vi "Read Lockinsens.vi"(1 "VISA resource name":refnum<visa-resource-name>="COM12", 2 "Voltage(T) Current(F)":bool=TRUE) -> (0 "Sensitivity":dbl=1e-08)   [LabVIEW 2013]
uses:
  <vilib>/Instr/_visa.llb/VISA Configure Serial Port (Instr).vi
panel:
  in  "milliseconds to wait":u32=50
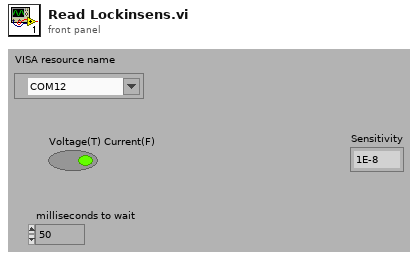
[diagram p1: front panel]
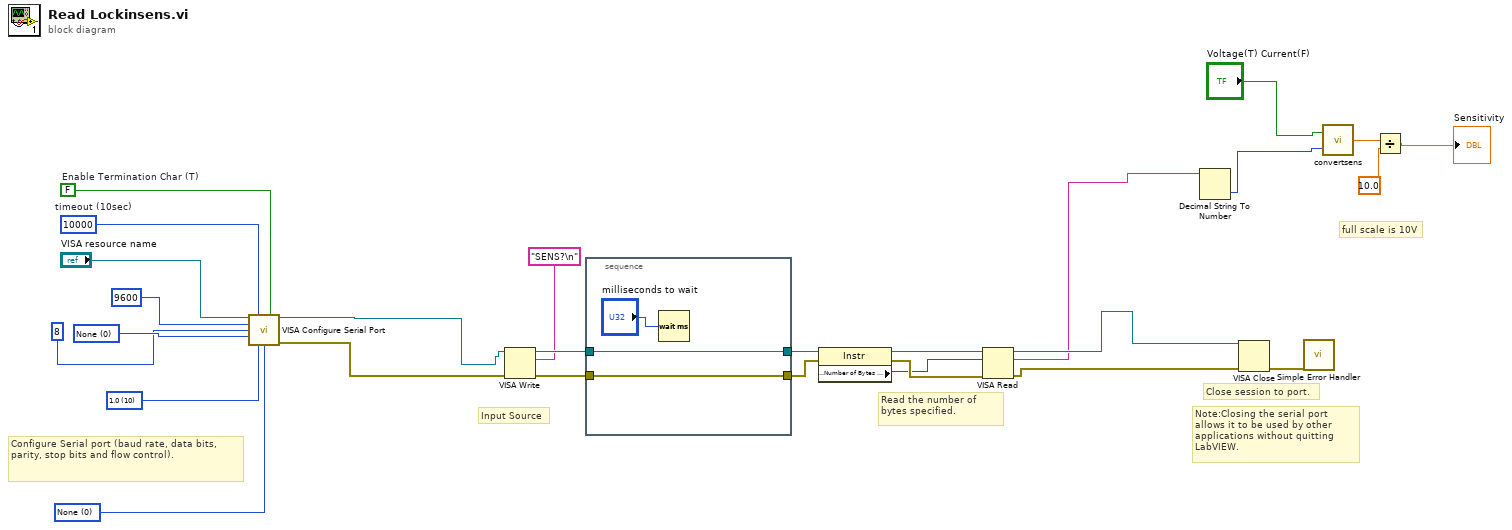
[diagram p0: block diagram]
diagram:
  w10 = u16 0 items=["None"=0, "XON/XOFF"=1, "RTS/CTS"=2, "DTR/DSR"=4] ("flow control")
  w11 = u16 10 items=["1.0"=10, "1.5"=15, "2.0"=20] ("stop bits")
  w14 = u16 0 items=["None", "Odd", "Even", "Mark", "Space"] ("parity")
  w12 = FALSE  # Enable Termination Char (T)
  w13 = u32 10000  # timeout (10sec)
  # "full scale is 10V"
  # "Configure Serial port (baud rate, data bits, parity, stop bits and flow control)."
  # "Input Source"
  # "Read the number of bytes specified."
  # "Note:Closing the serial port allows it to be used by other applications without quitting LabVIEW."
  # "Close session to port."
  n1 = call-poly "VISA Configure Serial Port"("VISA resource name"="VISA resource name", "timeout (10sec)"=w13, "Enable Termination\nChar (T)"=w12, "baud rate (9600)"=u32 9600 ("baud rate"), "data bits (8)"=u16 8 ("data bits"), "parity (0:none)"=w14, "stop bits (10: 1 bit)"=w11, "flow control (0:none)"=w10) -> ("VISA resource name out"=w7:refnum<visa-resource-name>, "error out"=w8:errorcluster)  [unwired: 1 in, 5 out]
  n2 = VISA Write(VISA resource name=w7, write buffer="SENS?\n" ("string to write"), error in (no error)=w8) -> (VISA resource name out=w22:refnum<visa-resource-name>, error out=w24:errorcluster)  [unwired: 1 out]
  n3 = stacked-sequence {
    tunnel: w24 -> [w30]
    tunnel: [w30] -> w23
    tunnel: w22 -> [w29]
    tunnel: [w29] -> w21
    frame #0 {
      n4 = Wait (ms)(milliseconds to wait="milliseconds to wait") -> ()  [unwired: 1 out]
    }
  }
  n5 = property class="Instr"(reference=w21, error in=w23) -> (reference out=w20:refnum<visa-resource-name>, error out=w19:errorcluster, "Serial Settings:Number of Bytes at Serial Port"=w18:u32)
  n6 = VISA Read(VISA resource name=w20, byte count=w18, error in (no error)=w19) -> (VISA resource name out=w26:refnum<visa-resource-name>, read buffer=w6:string, error out=w27:errorcluster)  [unwired: 1 out]
  n7 = Decimal String To Number(string=w6) -> (number=w4:i32)  [unwired: 2 in, 1 out]
  n8 = VISA Close(VISA resource name=w26, error in (no error)=w27) -> (error out=w25:errorcluster)
  n9 = call <vilib>:"Simple Error Handler.vi"("error in (no error)"=w25) -> ()  [unwired: 1 in, 8 out]
  n10 = call "convertsens.vi"("Lockin input"=w4, "Voltage(T) Current(F)"="Voltage(T) Current(F)") -> ("Sensitivity"=w3:dbl)
  n11 = Divide(x=w3, y=10.0) -> (x/y=→"Sensitivity":dbl)
